vi "counter_config.vi"(8 "error in (no error)":errorcluster, 9 "Nastaveni citace":T1, 10 "Kalibracni bod":T2, 11 "VISA Refnum in":refnum<visa-resource-name>) -> (0 "error out":errorcluster, 3 "VISA Refnum out":refnum<visa-resource-name>)   [LabVIEW 2022 SP3]
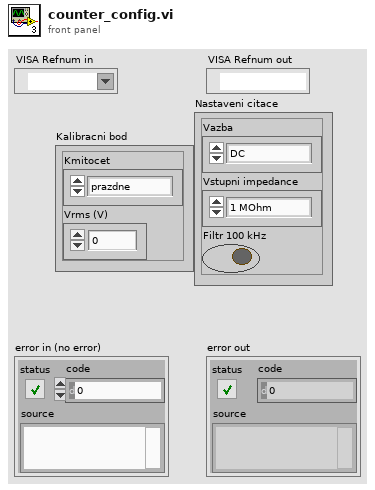
[diagram p1: front panel]
types:
  T1 = cluster{"Vazba":enum16{"DC", "AC"}, "Vstupni impedance":enum16{"1 MOhm", "50 Ohm"}, "Filtr 100 kHz":bool}
  T2 = cluster{"Kmitocet":enum16{"prazdne", "50 Hz", "1 kHz", "5 kHz", "10 kHz", "20 kHz", "50 kHz", "100 kHz"}, "Vrms (V)":dbl}
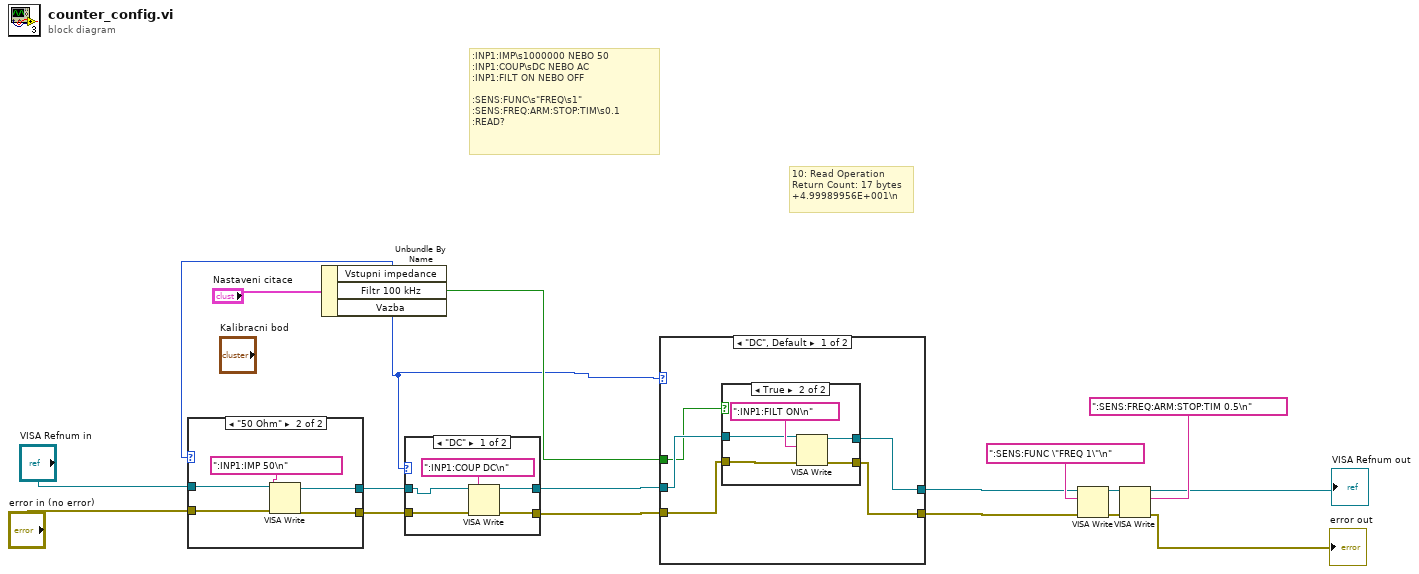
[diagram p0: block diagram]
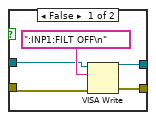
[diagram p2: hidden frame]
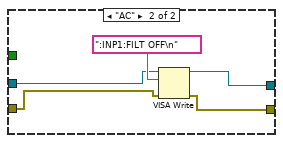
[diagram p3: hidden frame]
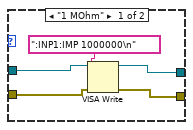
[diagram p4: hidden frame]
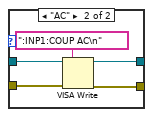
[diagram p5: hidden frame]
diagram:
  # "10: Read Operation\nReturn Count: 17 bytes\n+4.99989956E+001\\n"
  # ":INP1:IMP\\s1000000 NEBO 50\n:INP1:COUP\\sDC NEBO AC\n:INP1:FILT ON NEBO OFF\n\n:SENS:FUNC\\s\"FREQ\\s1\"\n:SENS:FREQ:ARM:STOP:TIM\\s0.1\n:READ?"
  n1 = Unbundle By Name("Nastaveni citace") -> ("Vstupni impedance"=w2:enum16{"1 MOhm", "50 Ohm"}, "Filtr 100 kHz"=w3:bool, "Vazba"=w1:enum16{"DC", "AC"})
  n2 = case shown="\"50 Ohm\"" w2 {
    tunnel: "error in (no error)" -> [w21 w27]
    tunnel: "VISA Refnum in" -> [w22 w26]
    tunnel: [w19 w25] -> w14
    tunnel: [w20 w24] -> w4
    frame "1 MOhm" {
      n3 = VISA Write(VISA resource name=w22, write buffer=":INP1:IMP 1000000\n", error in (no error)=w21) -> (VISA resource name out=w20:refnum<visa-resource-name>, error out=w19:errorcluster)  [unwired: 1 out]
    }
    frame "50 Ohm" {
      n4 = VISA Write(VISA resource name=w26, write buffer=":INP1:IMP 50\n", error in (no error)=w27) -> (VISA resource name out=w24:refnum<visa-resource-name>, error out=w25:errorcluster)  [unwired: 1 out]
    }
  }
  n5 = case shown="\"DC\"" w1 {
    tunnel: w4 -> [w32 w37]
    tunnel: w14 -> [w31 w36]
    tunnel: [w29 w35] -> w13
    tunnel: [w30 w34] -> w12
    frame "DC" {
      n6 = VISA Write(VISA resource name=w32, write buffer=":INP1:COUP DC\n", error in (no error)=w31) -> (VISA resource name out=w29:refnum<visa-resource-name>, error out=w30:errorcluster)  [unwired: 1 out]
    }
    frame "AC" {
      n7 = VISA Write(VISA resource name=w37, write buffer=":INP1:COUP AC\n", error in (no error)=w36) -> (VISA resource name out=w35:refnum<visa-resource-name>, error out=w34:errorcluster)  [unwired: 1 out]
    }
  }
  n8 = case shown="\"DC\", Default" w1 {
    tunnel: w13 -> [w42 w56]
    tunnel: w12 -> [w43 w57]
    tunnel: [w40 w55] -> w11
    tunnel: [w41 w54] -> w10
    tunnel: w3 -> [w39 _]
    frame "DC", Default {
      n9 = case shown="True" w39 {
        tunnel: w42 -> [w46 w52]
        tunnel: w43 -> [w47 w51]
        tunnel: [w45 w50] -> w40
        tunnel: [w44 w49] -> w41
        frame False {
          n10 = VISA Write(VISA resource name=w46, write buffer=":INP1:FILT OFF\n", error in (no error)=w47) -> (VISA resource name out=w45:refnum<visa-resource-name>, error out=w44:errorcluster)  [unwired: 1 out]
        }
        frame True {
          n11 = VISA Write(VISA resource name=w52, write buffer=":INP1:FILT ON\n", error in (no error)=w51) -> (VISA resource name out=w50:refnum<visa-resource-name>, error out=w49:errorcluster)  [unwired: 1 out]
        }
      }
    }
    frame "AC" {
      n12 = VISA Write(VISA resource name=w56, write buffer=":INP1:FILT OFF\n", error in (no error)=w57) -> (VISA resource name out=w55:refnum<visa-resource-name>, error out=w54:errorcluster)  [unwired: 1 out]
    }
  }
  n13 = VISA Write(VISA resource name=w11, write buffer=":SENS:FUNC \"FREQ 1\"\n", error in (no error)=w10) -> (VISA resource name out=w9:refnum<visa-resource-name>, error out=w8:errorcluster)  [unwired: 1 out]
  n14 = VISA Write(VISA resource name=w9, write buffer=":SENS:FREQ:ARM:STOP:TIM 0.5\n", error in (no error)=w8) -> (VISA resource name out=→"VISA Refnum out":refnum<visa-resource-name>, error out=→"error out":errorcluster)  [unwired: 1 out]
